vi "Map Extension Examples.vi"() -> ()   [LabVIEW 2020]
uses:
  d52ac117-3a0c-4c38-a035-cd1ec790ca6a.vi
  158e93f0-6d83-44df-a97f-fd033c23c3c4.vi
  75fe9182-0039-4258-ba56-e63b77652130.vi
  0236d640-7fb0-4049-b526-a4a0acec0d8d.vi
  77e0272d-242f-412b-982f-1600aba21800.vi
  8d18f84e-651b-4bc2-8d26-9827fa866315.vi
  332644c8-09cd-45c9-9348-425bf23ac390.vi
  14195457-9666-4654-9939-676a4b3105cd.vi
  75fe9182-0039-4258-ba56-e63b77652130.vi/b0178052-0c48-4c9a-874f-40b592e34ac5.vi
  77e0272d-242f-412b-982f-1600aba21800.vi/8ee94aa7-4836-4e87-a0a7-557d81cff62b.vi
panel:
  out "key found?":bool
  out "Created Empty Map?":bool
  out "keys":string[](array[string])
  out "Keys":i32[](array[numeric])
  out "Converted Array to Map?":bool
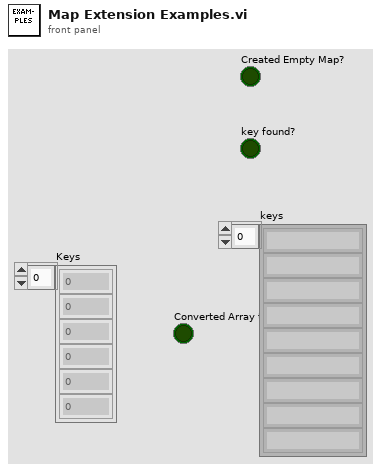
[diagram p1: front panel]
types:
  T1 = cluster{"bool":bool, "string":string, "bool 2":bool, "Name":i32}
  T2 = map{string, cluster{"bool":bool, "string":string, "bool 2":bool, "Name":i32}}
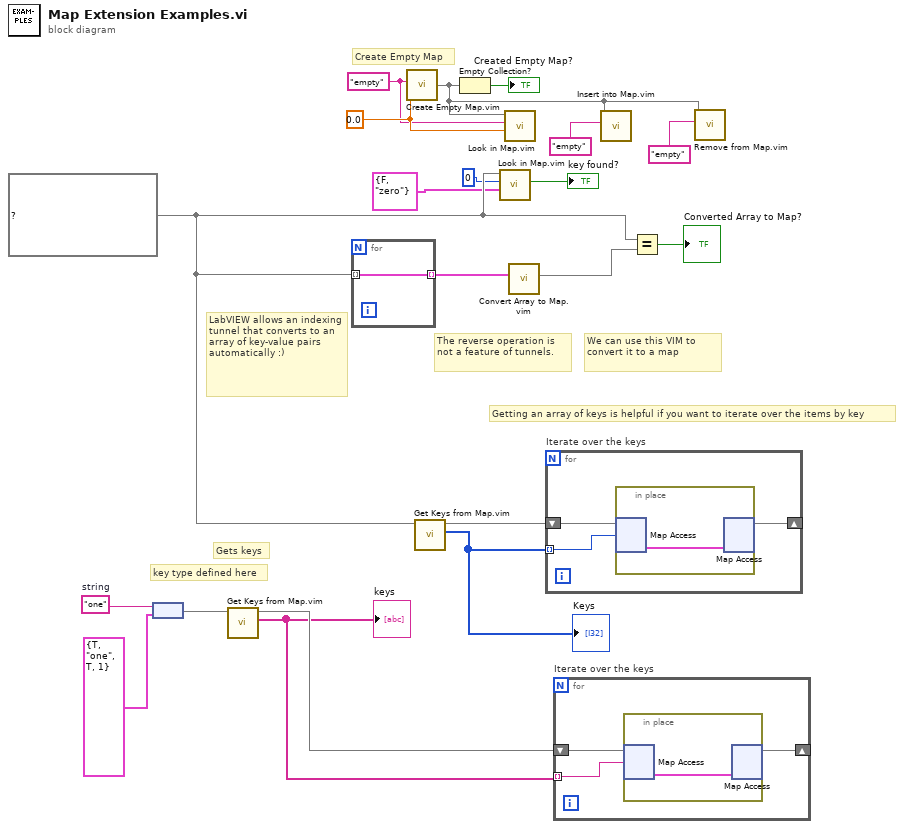
[diagram p0: block diagram]
diagram:
  w7 = map{i32, cluster{"bool":bool, "string":string}} {0={"bool"=FALSE, "string"="zero"}, 1={"bool"=TRUE, "string"="one"}} ("map out")
  w8 = 0.0
  w4 = "empty" ("key type")
  w14 = "one"  # string
  # "Getting an array of keys is helpful if you want to iterate over the items by key"
  # "key type defined here"
  # "Gets keys"
  # "We can use this VIM to convert it to a map"
  # "The reverse operation is not a feature of tunnels."
  # "Create Empty Map"
  # "LabVIEW allows an indexing tunnel that converts to an array of key-value pairs automatically :)"
  n1 = node(w14, T1 {"bool"=TRUE, "string"="one", "bool 2"=TRUE, "Name"=1}) -> (w13:T2)
  n2 = call "Get Keys from Map.vim"("map"=w13) -> ("keys"=w10:string[], "map out"=w11:T2)  [unwired: 9 in]
  "keys" <- w10
  n3 = for {
    tunnel: [w21] -> w20 mode=indexing
    tunnel: w7 -> [w21] mode=indexing
  }
  n4 = call "Create Empty Map.vim"("value type"=w8, "key type"=w4) -> ("empty map"=w2:map{string, dbl})  [unwired: 8 in]
  n5 = call "Get Keys from Map.vim"("map"=w7) -> ("keys"=w17:i32[], "map out"=w16:map{i32, cluster{"bool":bool, "string":string}})  [unwired: 9 in]
  "Keys" <- w17
  n6 = Empty Collection?(1:w2) -> (0:→"Created Empty Map?":bool)
  n7 = call "Look in Map.vim"("default value"=cluster{"bool":bool, "string":string} {"bool"=FALSE, "string"="zero"} ("value"), "key"=0 ("Name"), "map"=w7) -> ("key found?"=→"key found?":bool)  [unwired: 7 in, 1 out]
  n8 = call "Look in Map.vim"("default value"=w8, "key"=w4, "map"=w2) -> ()  [unwired: 7 in, 2 out]
  n9 = call "Convert Array to Map.vim"("array"=w20) -> ("map"=w19:map{i32, cluster{"bool":bool, "string":string}})  [unwired: 10 in]
  n10 = for "Iterate over the keys" {
    shift-right: [w22] -> _
    shift-left: w16 -> [w23]
    tunnel: w17 -> [w24] mode=indexing
    n11 = in-place {
      n12 = in-place-map #1(w23, w24) -> (w25:cluster{"bool":bool, "string":string})  [unwired: 1 in, 1 out]
      n13 = in-place-map #1(w25) -> (w22:map{i32, cluster{"bool":bool, "string":string}})  [unwired: 1 in, 2 out]
    }
  }
  n14 = for "Iterate over the keys" {
    shift-right: [w26] -> _
    shift-left: w11 -> [w27]
    tunnel: w10 -> [w28] mode=indexing
    n15 = in-place {
      n16 = in-place-map #2(w27, w28) -> (w29:T1)  [unwired: 1 in, 1 out]
      n17 = in-place-map #2(w29) -> (w26:T2)  [unwired: 1 in, 2 out]
    }
  }
  n18 = call "Insert into Map.vim"("key"="empty" ("key type"), "map"=w2) -> ()  [unwired: 7 in, 3 out]
  n19 = Equal?(x=w7, y=w19) -> (x = y?=→"Converted Array to Map?":bool)
  n20 = call "Remove from Map.vim"("key"="empty" ("key type"), "map"=w2) -> ()  [unwired: 7 in, 3 out]
